vi "20200306_DynamicAndStatic_Final.vi"() -> ()   [LabVIEW 2020]
uses:
  Test Case Control.ctl
  <vilib>/Instr/_visa.llb/VISA Open Access Mode.ctl
  <vilib>/Platform/TimedLoop/XDataNode/timing_clust.ctl
  <vilib>/Platform/TimedLoop/XDataNode/nitl_modes.ctl
  <vilib>/Platform/TimedLoop/XDataNode/wakeup.ctl
  <vilib>/Analysis/baseanly.llb/Mean (DBL).vi
  <vilib>/Instr/_visa.llb/VISA Configure Serial Port (Instr).vi
  <vilib>/platform/TimedLoop/XDataNode/XDataNode.xnode
  <vilib>/Analysis/NI_AALBase.lvlib
  <vilib>/Platform/TimedLoop/XDataNode/XDNodeRunTimeDep.lvlib
panel:
  in  "?":bool
  out "Dynamic LF":dbl
  out "Static LF":dbl
  in  "?":enum32{"Hand Device GUI"}(tab)
  in  "Trial":string="1"
  in  "Weight Applied (g)":enum16{"0", "450"}(ring)
  in  "Group ID":enum16{"1", "2"}(ring)
  in  "Hand in Test":enum16{"Right", "Left"}(ring)
  in  "Time between beeps (ms)":dbl=3500.0
  in  "Test Case":T1
  out "Grip Force":dynamicdata(graph)
  in  "Exit":bool
  out "Calibration Complete":bool
  in  "Calibrate System\nButton":bool
  in  "Calibration Time (ms)":dbl=3000.0 caption="Time Target (s)"
  in  "Patient ID":string="1"
  in  "File Path":path=path "C:/Users/rsKite/Documents/Data_logs"
  in  "COM Port":refnum<visa-resource-name>="COM3"
  in  "Start Collecting":bool
  out "Load Force":dynamicdata(graph)
  out "Dynamic Flag":i32
  in  "Wait Time Before Starting Test (ms)":u32=3000
  out "error out":errorcluster
  # "____________ Calibration ____________"
  # "____________ Test Setup ____________"
  # "(Dynamic Case ONLY)"
  # "________ Patient Information ________"
  # "_________ Data Collection _________"
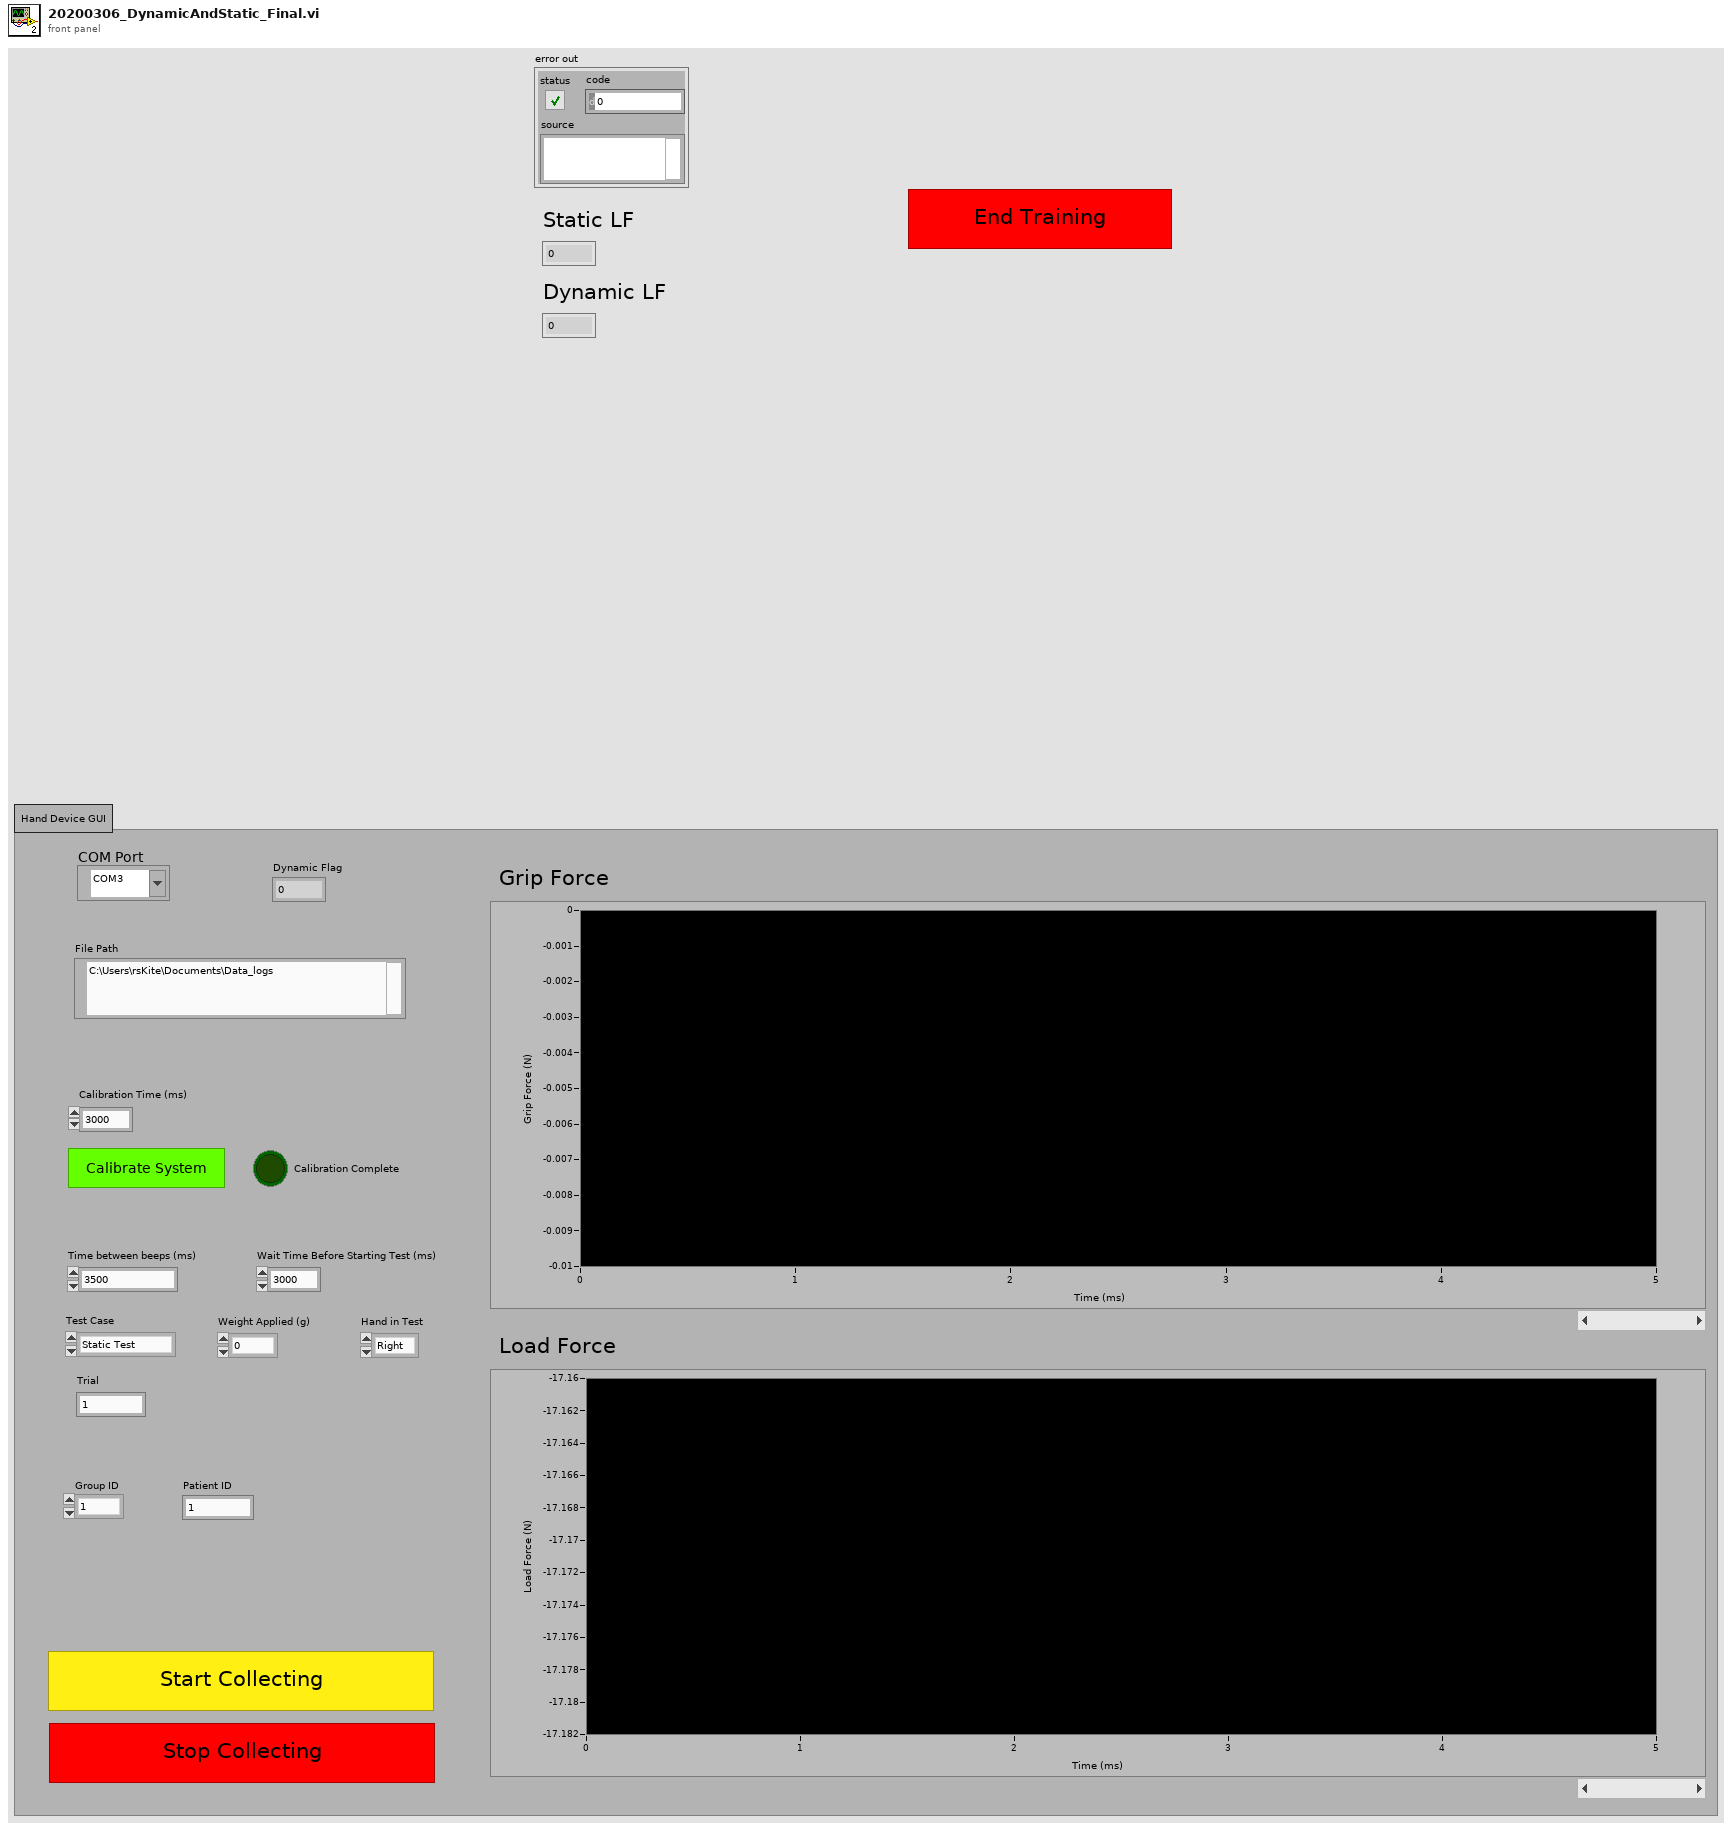
[diagram p1: front panel]
types:
  T1 = typedef "Test Case Control.ctl" = enum16{"Static Test", "Dynamic Test"}
  T2 = typedef "XDNodeRunTimeDep.lvlib/timing_clust.ctl" = cluster{"Expected End [f-1]":u64, "Actual End [f-1]":u64, "Finished Late? [f-1]":bool, "Expected End [i-1]":u64, "Actual End [i-1]":u64, "Finished Late? [i-1]":bool, "Expected Start [i]":u64, "Actual Start [i]":u64, "Expected Start [f]":u64, "Actual Start [f]":u64, "Source Name":string, "Structure Name":string, "Period":i64, "Deadline":i64, "Offset":i64, "Start":i64, "Priority":i32, "Timeout":i32, "Mode":T3, "Wakeup Reason":T4, "Error":errorcluster, "Source Type":string, "Secondary Source Type":string, "Global End Time":u64, "Global Start Time":u64, "Frame Duration":u64, "Iteration Duration":u64, "Assigned CPU":i32, "I/O Scan Engine Mode":u32}
  T3 = typedef "XDNodeRunTimeDep.lvlib/nitl_modes.ctl" = enum32{"No Change", "Process missed periods, maintain original phase", "Discard missed periods, maintain original phase", "Process missed periods, ignore original phase", "Discard missed periods, ignore original phase"}
  T4 = typedef "XDNodeRunTimeDep.lvlib/wakeup.ctl" = enum32{"Normal", "Aborted", "Asynchronous wakeup", "Timing source error", "Timed loop error", "Timeout"}
  T5 = enum16{"open", "replace", "create", "open or create", "replace or create", "replace or create with confirmation"}
  T6 = typedef "VISA Open Access Mode.ctl" = u32
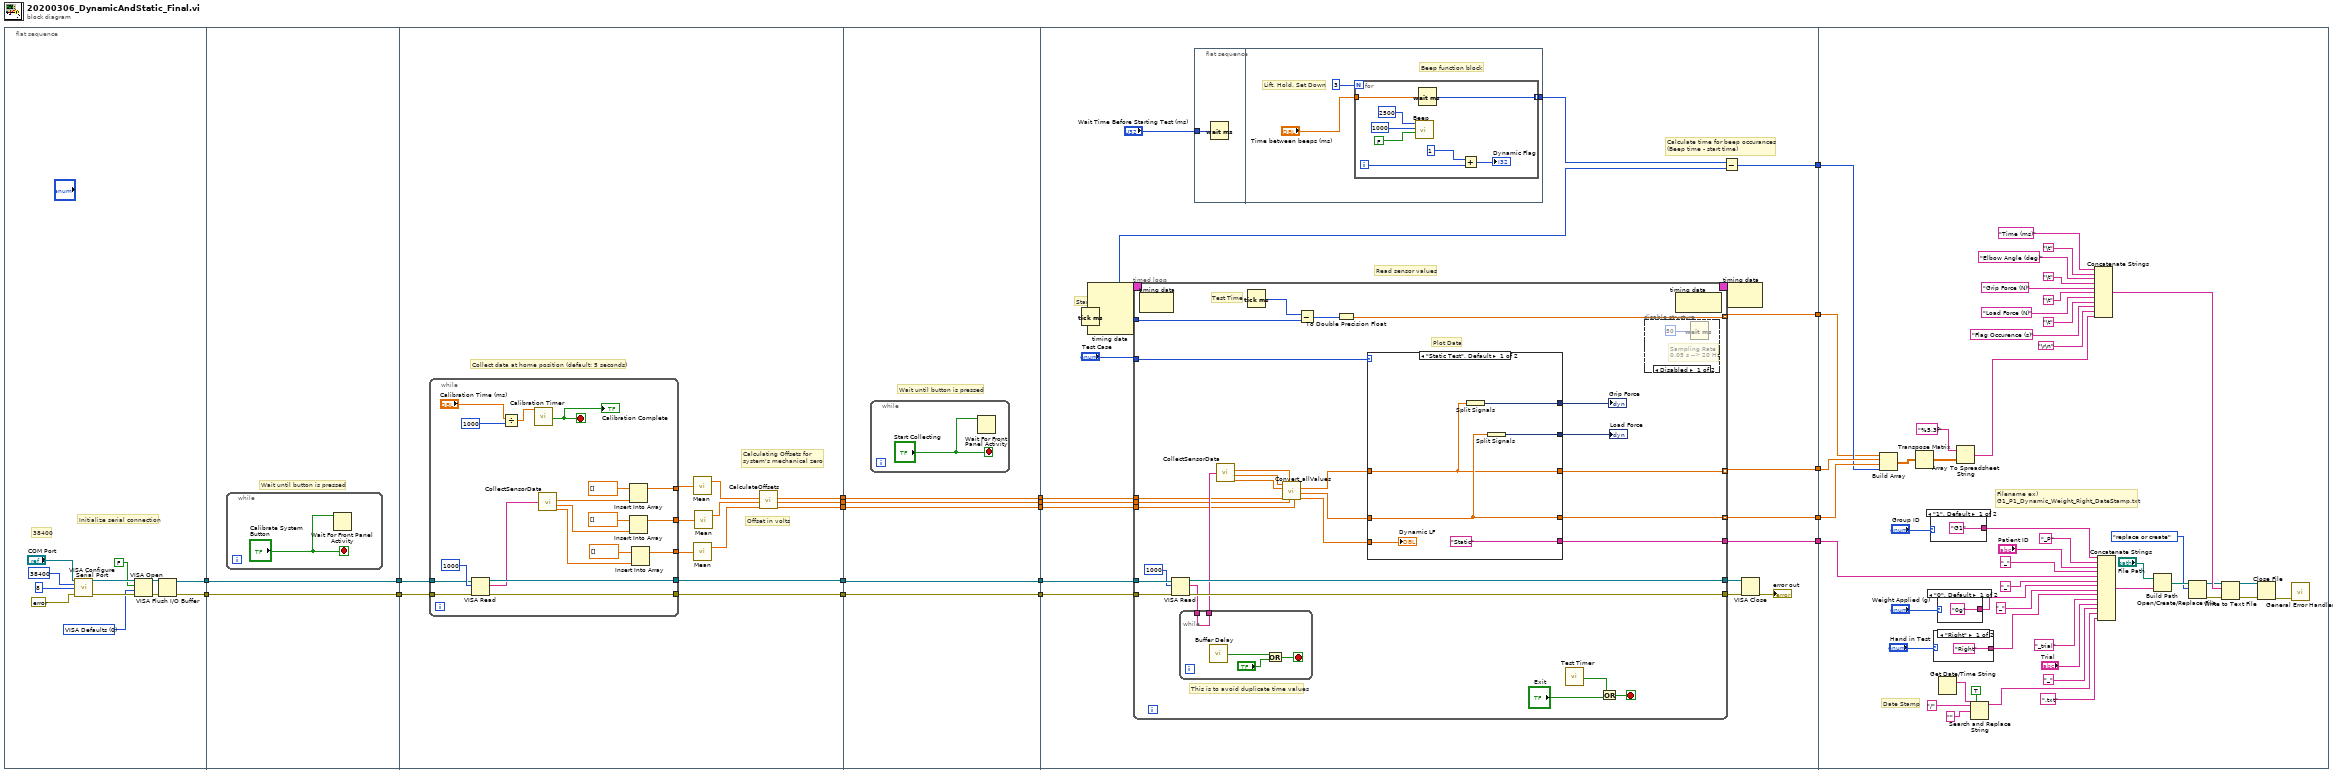
[diagram p0: block diagram]
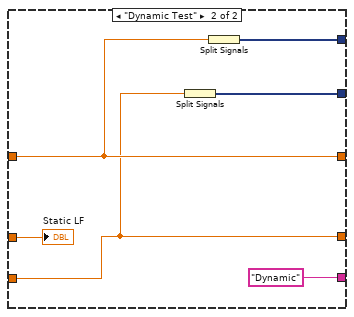
[diagram p3: hidden frame]
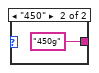
[diagram p4: hidden frame]
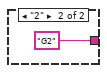
[diagram p5: hidden frame]
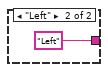
[diagram p6: hidden frame]
diagram:
  n1 = flat-sequence {
    tunnel: [w23] -> w19
    tunnel: [w22] -> w18
    tunnel: w19 -> [w33]
    tunnel: [w33] -> w17
    tunnel: w18 -> [w32]
    tunnel: [w32] -> w16
    tunnel: w17 -> [w47]
    tunnel: [w44] -> w15
    tunnel: w16 -> [w46]
    tunnel: [w45] -> w14
    tunnel: [w37] -> w13
    tunnel: [w36] -> w12
    tunnel: [w35] -> w11
    tunnel: w15 -> [w71]
    tunnel: [w71] -> w10
    tunnel: w14 -> [w70]
    tunnel: [w70] -> w9
    tunnel: w13 -> [w69]
    tunnel: [w69] -> w8
    tunnel: w12 -> [w68]
    tunnel: [w68] -> w7
    tunnel: w11 -> [w67]
    tunnel: [w67] -> w6
    tunnel: w10 -> [w90]
    tunnel: w9 -> [w89]
    tunnel: w8 -> [w85]
    tunnel: w7 -> [w84]
    tunnel: w6 -> [w83]
    tunnel: [w82] -> w5
    tunnel: [w81] -> w4
    tunnel: [w80] -> w3
    tunnel: [w79] -> w2
    tunnel: [w78] -> w1
    tunnel: w5 -> [w165]
    tunnel: w4 -> [w154]
    tunnel: w3 -> [w177]
    tunnel: w2 -> [w171]
    tunnel: w1 -> [w170]
    frame #0 {
      w21 = T6 0 items=["VISA Defaults"=0, "Exclusive Lock"=1, "Load Configured Settings"=4] ("Access Mode")
      # "38400"
      # "Initialize serial connection"
      n2 = call-poly "VISA Configure Serial Port"("VISA resource name"="COM Port", "baud rate (9600)"=u32 38400, "data bits (8)"=u16 8, "error in (no error)"=errorcluster {"status"=FALSE, "code"=0, "source"=""}) -> ("VISA resource name out"=w29:refnum<visa-resource-name>, "error out"=w27:errorcluster)  [unwired: 10 in]
      n3 = VISA Open(duplicate session (F)=FALSE, access mode=w21, error in (no error)=w27, VISA resource name=w29) -> (VISA resource name=w30:refnum<visa-resource-name>, error out=w31:errorcluster)  [unwired: 1 in]
      n4 = VISA Flush I/O Buffer(VISA resource name=w30, error in (no error)=w31) -> (VISA resource name out=w22:refnum<visa-resource-name>, error out=w23:errorcluster)  [unwired: 1 in]
    }
    frame #1 {
      # "Wait until button is pressed"
      n5 = while {
        stop <- "Calibrate System\nButton" stop-if-true
        n6 = Wait For Front Panel Activity(3:"Calibrate System\nButton") -> ()  [unwired: 2 in, 1 out]
      }
    }
    frame #2 {
      # "Offset in volts"
      # "Calculating Offsets for\nsystem's mechanical zero"
      # "Collect data at home position (default: 5 seconds)"
      n7 = while {
        tunnel: w47 -> [w65]
        tunnel: w46 -> [w64]
        tunnel: [w63] -> w45
        tunnel: [w62] -> w44
        tunnel: [w61] -> w43
        tunnel: [w60] -> w42
        tunnel: [w55] -> w41
        stop <- w57 stop-if-true
        n8 = VISA Read(VISA resource name=w64, byte count=u32 1000, error in (no error)=w65) -> (VISA resource name out=w63:refnum<visa-resource-name>, read buffer=w52:string, error out=w62:errorcluster)  [unwired: 1 out]
        n9 = Divide(x="Calibration Time (ms)", y=1000) -> (x/y=w48:dbl)
        n10 = call "Calibration Timer"("Time Target (s)"=w48) -> ("Time has Elapsed"=w57:bool)  [unwired: 11 in, 7 out]
        "Calibration Complete" <- w57
        n11 = call "CollectSensorData.vi"("Serial buffer"=w52) -> ("Grip Force"=w54:dbl, "Static Futek Volts"=w53:dbl, "Dynamic Load Force"=w51:dbl)  [unwired: 1 in]
        n12 = Insert Into Array(array=dbl[] [], new element=w54) -> (w60:dbl[])  [unwired: 1 in]
        n13 = Insert Into Array(array=dbl[] [], new element=w53) -> (w55:dbl[])  [unwired: 1 in]
        n14 = Insert Into Array(array=dbl[] [], new element=w51) -> (w61:dbl[])  [unwired: 1 in]
      }
      n15 = call-poly <vilib>:"Mean.vi"("X"=w42) -> ("mean"=w39:dbl)  [unwired: 1 out]
      n16 = call-poly <vilib>:"Mean.vi"("X"=w43) -> ("mean"=w38:dbl)  [unwired: 1 out]
      n17 = call-poly <vilib>:"Mean.vi"("X"=w41) -> ("mean"=w40:dbl)  [unwired: 1 out]
      n18 = call "CalculateOffsets.vi"("Dynamic LF"=w38, "Static LF"=w40, "GF"=w39) -> ("Dynamic LF Offset"=w37:dbl, "Static LF Offset"=w36:dbl, "GF Offset"=w35:dbl)  [unwired: 2 in]
    }
    frame #3 {
      # "Wait until button is pressed"
      n19 = while {
        stop <- "Start Collecting" stop-if-true
        n20 = Wait For Front Panel Activity(3:"Start Collecting") -> ()  [unwired: 2 in, 1 out]
      }
    }
    frame #4 {
      # "Read sensor values"
      # "Calculate time for beep occurances\n(Beep time - start time)"
      # "Start Time"
      n21 = Tick Count (ms)() -> (millisecond timer value=w75:u32)
      n22 = node-c288() -> (w74:T2)  [unwired: 4 in]
      n23 = timed-loop {
        tunnel: w90 -> [w118]
        tunnel: w89 -> [w117]
        tunnel: [w114] -> w88
        tunnel: [w113] -> w87
        tunnel: "Test Case" -> [w112]
        tunnel: w75 -> [w111]
        tunnel: w85 -> [w95]
        tunnel: w84 -> [w96]
        tunnel: w83 -> [w97]
        tunnel: [w107] -> w82
        tunnel: [w105] -> w81 mode=indexing
        tunnel: [w103] -> w80 mode=indexing
        tunnel: [w104] -> w79 mode=indexing
        timing: w74 -> [_]
        timing-out: [_] -> w73
        stop <- w108 stop-if-true
        # "This is to avoid duplicate time values"
        # "Plot Data"
        # "Test Time"
        n24 = node-c288() -> ()  [unwired: 1 in, 1 out]
        n25 = VISA Read(VISA resource name=w117, byte count=u32 1000, error in (no error)=w118) -> (VISA resource name out=w114:refnum<visa-resource-name>, read buffer=w110:string, error out=w113:errorcluster)  [unwired: 1 out]
        n26 = while {
          tunnel: w110 -> [w124]
          tunnel: [w124] -> w101
          stop <- w125 stop-if-true
          n27 = call "Buffer Delay"() -> ("Time has Elapsed"=w126:bool)  [unwired: 12 in, 7 out]
          n28 = Or(x=w126, y="?") -> (x .or. y?=w125:bool)
        }
        n29 = call "CollectSensorData.vi"("Serial buffer"=w101) -> ("Grip Force"=w100:dbl, "Static Futek Volts"=w99:dbl, "Dynamic Load Force"=w98:dbl)  [unwired: 1 in]
        n30 = Tick Count (ms)() -> (millisecond timer value=w119:u32)
        n31 = call "Convert_allValues.vi"("Accel (MPU6050) Offset"=w95, "Load (Futek) Offset"=w96, "Grip (Omega) Value"=w100, "Grip (Omega) Offset"=w97, "Accel (MPU6050) Value"=w98, "Load (Futek) Value"=w99) -> ("Dynamic Load Force"=w92:dbl, "Static Load Force"=w93:dbl, "Grip Force"=w94:dbl)  [unwired: 3 in]
        n32 = Subtract(x=w119, y=w111) -> (x-y=w106:u32)
        n33 = To Double Precision Float(number=w106) -> (double precision float=w105:dbl)
        n34 = case shown="\"Static Test\", Default" w112 {
          tunnel: [w131 w135] -> w104
          tunnel: [w130 w136] -> w103
          tunnel: [w129 w137] -> w116
          tunnel: ["Static" "Dynamic"] -> w107
          tunnel: w94 -> [w130 w136]
          tunnel: w93 -> [w131 w138]
          tunnel: w92 -> [w132 w135]
          tunnel: [w128 w134] -> w102
          frame "Static Test", Default {
            n35 = Split Signals(w130) -> (w129:dynamicdata)  [unwired: 1 in]
            n36 = Split Signals(w131) -> (w128:dynamicdata)  [unwired: 1 in]
            "Dynamic LF" <- w132
          }
          frame "Dynamic Test" {
            n37 = Split Signals(w135) -> (w134:dynamicdata)  [unwired: 1 in]
            n38 = Split Signals(w136) -> (w137:dynamicdata)  [unwired: 1 in]
            "Static LF" <- w138
          }
        }
        "Grip Force" <- w116
        "Load Force" <- w102
        n39 = call "Test Timer"() -> ("Time has Elapsed"=w120:bool)  [unwired: 12 in, 7 out]
        n40 = Or(x=w120, y="Exit") -> (x .or. y?=w108:bool)
        n41 = disable-structure shown="Disabled" {
          frame Disabled {
            # "Sampling Rate\n0.05 s --> 20 Hz"
            n42 = Wait (ms)(milliseconds to wait=u32 50) -> ()  [unwired: 1 out]
          }
          frame Enabled {
          }
        }
        n43 = node-c288() -> ()  [unwired: 1 in, 1 out]
      }
      n44 = flat-sequence {
        tunnel: "Wait Time Before Starting Test (ms)" -> [w142]
        tunnel: [w143] -> w76
        frame #0 {
          n45 = Wait (ms)(milliseconds to wait=w142) -> ()  [unwired: 1 out]
        }
        frame #1 {
          # "Beep function block"
          # "Lift, Hold, Set Down"
          n46 = for {
            N: 3 -> [_]
            tunnel: "Time between beeps (ms)" -> [w150]
            tunnel: [w146] -> w143 mode=indexing
            i -> [w149]
            n47 = call <vilib>:"Beep.vi"("use system alert? (T)"=FALSE, "duration (msec)"=u32 1000, "frequency (Hz)"=u32 2500) -> ()  [unwired: 9 in]
            n48 = Wait (ms)(milliseconds to wait=w150) -> (millisecond timer value=w146:u32)
            n49 = Add(x=1, y=w149) -> (x+y=→"Dynamic Flag":i32)
          }
        }
      }
      n50 = Subtract(x=w76, y=w75) -> (x-y=w78:u32[])
      n51 = node-c288(w73) -> ()  [unwired: 1 out]
      n52 = VISA Close(VISA resource name=w88, error in (no error)=w87) -> (error out=→"error out":errorcluster)
    }
    frame #5 {
      # "Filename ex)\nG1_P1_Dynamic_Weight_Right_DateStamp.txt"
      # "Date Stamp"
      n53 = Build Array(w154, w177, w171, w170) -> (w176:dbl[][])
      n54 = Transpose Matrix(1:w176) -> (0:w192:dbl[][])
      n55 = case shown="\"1\", Default" "Group ID" {
        tunnel: ["G1" "G2"] -> w167
        frame "1", Default {
        }
        frame "2" {
        }
      }
      n56 = case shown="\"Right\"" "Hand in Test" {
        tunnel: ["Right" "Left"] -> w162
        frame "Right" {
        }
        frame "Left" {
        }
      }
      n57 = case shown="\"0\", Default" "Weight Applied (g)" {
        tunnel: ["0g" "450g"] -> w160
        frame "0", Default {
        }
        frame "450" {
        }
      }
      n58 = Get Date/Time String() -> (date string=w201:string)  [unwired: 3 in, 1 out]
      n59 = Array To Spreadsheet String(array=w192, 3:"%5.3f" ("format string")) -> (spreadsheet string=w175:string)  [unwired: 1 in]
      n60 = Search and Replace String(replace all?=TRUE ("replace all? (F)"), input string=w201, search string="/", replace string="" ("replace string (\"\")")) -> (result string=w157:string)  [unwired: 4 in, 3 out]
      n61 = Concatenate Strings("Time (ms)" ("string"), "\t", "Elbow Angle (deg)" ("string"), "\t", "Grip Force (N)" ("string"), "\t", "Load Force (N)" ("string"), "\t", "Flag Occurence (s)", "\r\n", w175) -> (w202:string)
      n62 = Concatenate Strings(w167, "_P" ("string"), "Patient ID", "_" ("string"), w165, "_" ("string"), w160, "_" ("string"), w162, "_trial" ("string"), "Trial", "_" ("string"), w157, ".txt" ("string")) -> (w200:string)
      n63 = Build Path(base path="File Path", name or relative path=w200) -> (appended path=w199:path)
      n64 = Open/Create/Replace File(file path (use dialog)=w199, operation (0:open)=T5."replace or create") -> (refnum out=w193:refnum<file>, error out=w195:errorcluster)  [unwired: 4 in, 1 out]
      n65 = Write to Text File(file (use dialog)=w193, text=w202, error in=w195) -> (refnum out=w194:refnum<file>, error out=w196:errorcluster)  [unwired: 1 in, 1 out]
      n66 = Close File(refnum=w194, error in=w196) -> (error out=w197:errorcluster)  [unwired: 1 out]
      n67 = call <vilib>:"General Error Handler.vi"("error in (no error)"=w197) -> ()  [unwired: 10 in, 5 out]
    }
  }
